vi "Create Node.vi"(8 "error in (no error)":errorcluster, 9 "Display Name":string, 10 "UID":string, 11 "Base Tree in":refnum<class "Base Tree.lvclass">) -> (0 "error out":errorcluster, 3 "Base Tree out":refnum<class "Base Tree.lvclass">)   [LabVIEW 2017, in "opcua.lvlib" / "Browser Core.lvlib" / "Base Tree.lvclass"]
doc: "Create new Node and Add to Tree dictionary"
uses:
  Base Tree.lvclass
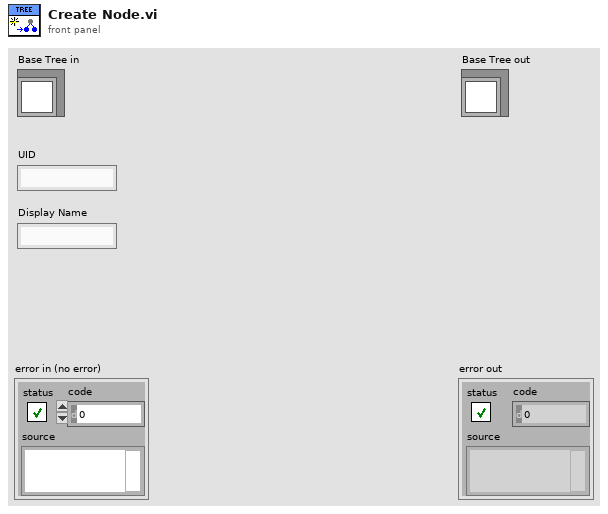
[diagram p1: front panel]
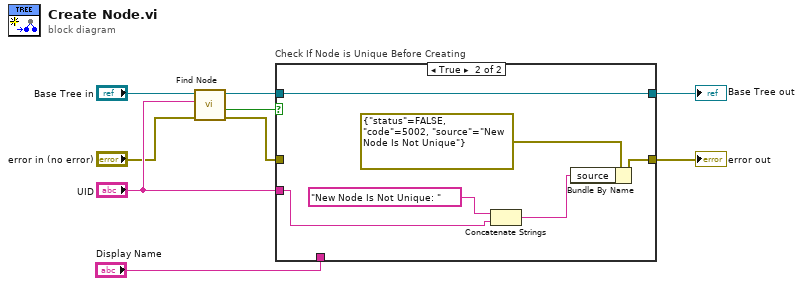
[diagram p0: block diagram]
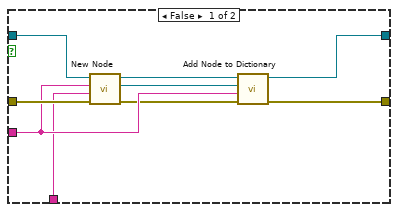
[diagram p2: hidden frame]
diagram:
  n1 = call-dynamic "Find Node.vi"("error in (no error)"="error in (no error)", "UID"="UID", "Base Tree in"="Base Tree in") -> ("error out"=w5:errorcluster, "Found?"=w6:bool, "Base Tree out"=w4:refnum<class "Base Tree.lvclass">)  [unwired: 5 in, 1 out]
  n2 = case "Check If Node is Unique Before Creating" shown="True" w6 {
    tunnel: "UID" -> [w14 w20]
    tunnel: w5 -> [w17 _]
    tunnel: w4 -> [w16 w23]
    tunnel: [w13 w19] -> w3
    tunnel: [w12 w23] -> w2
    tunnel: "Display Name" -> [w10 _]
    frame False {
      n3 = call-dynamic "New Node.vi"("error in (no error)"=w17, "Display Name"=w10, "UID"=w14, "Base Tree in"=w16) -> ("error out"=w13:errorcluster, "Generic Node out"=w11:refnum<class "Generic Node.lvclass">, "Base Tree out"=w15:refnum<class "Base Tree.lvclass">)  [unwired: 5 in]
      n4 = call "Add Node to Dictionary.vi"("Error In"=w13, "UID"=w14, "New Node"=w11, "Base Tree in"=w15) -> ("Base Tree out"=w12:refnum<class "Base Tree.lvclass">)  [unwired: 7 in]
    }
    frame True {
      n5 = Concatenate Strings("New Node Is Not Unique: " ("source"), w20) -> (w18:string)
      n6 = Bundle By Name(cluster=errorcluster {"status"=FALSE, "code"=5002, "source"="New Node Is Not Unique"} ("error out"), "source"=w18) -> (w19:errorcluster)
    }
  }
  "error out" <- w3
  "Base Tree out" <- w2
